vi "ZMQ.global.vi"() -> ()   [LabVIEW 2014]
uses:
  <vilib>/addons/zeromq/zmq_context.lvclass
  <vilib>/addons/zeromq/zmq_socket.lvclass
panel:
  out "ZMQ":T1
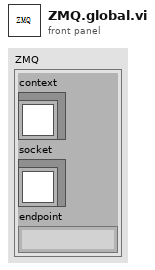
[diagram p1: front panel]
types:
  T1 = cluster{"context":refnum<class "zmq_context.lvclass">, "socket":refnum<class "zmq_socket.lvclass">, "endpoint":string}
diagram:
